vi "Send serial command.vi"(7 "Read?":bool, 8 "error IO":errorcluster, 10 "Send string":string=" 2 np", 11 "VISA resource name out":refnum<visa-resource-name>) -> (0 "error out":errorcluster={"status"=FALSE, "code"=1073676294, "source"="VISA Read in SMAC Parameters.vi->SMAC LabVIEW Toolkit_v1.vi"}, 2 "read string":string, 3 "VISA Out":refnum<visa-resource-name>)   [LabVIEW 2016]
panel:
  out "actual bytes read":u32
  out "Format String":string=" 1 03"
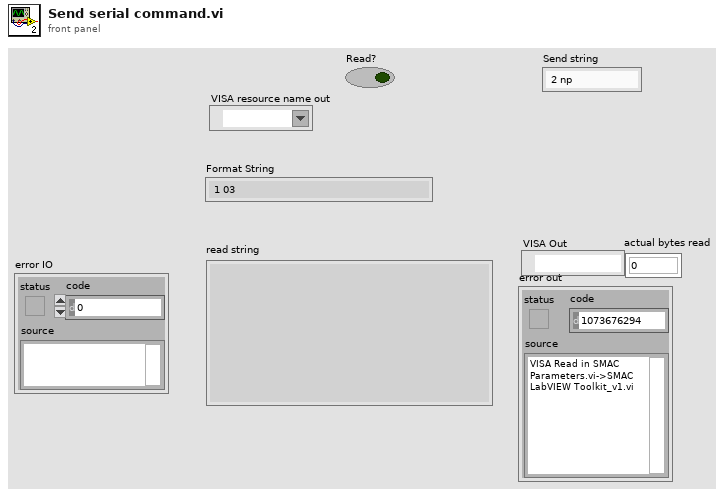
[diagram p1: front panel]
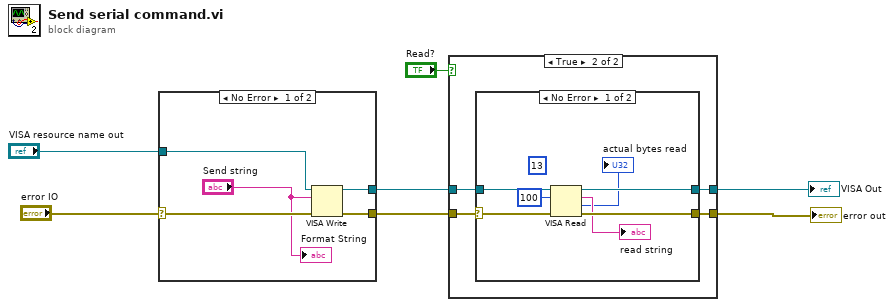
[diagram p0: block diagram]
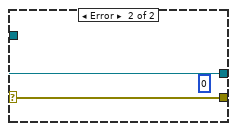
[diagram p4: hidden frame]
diagram:
  n1 = case shown="No Error" "error IO" {
    selector: "error IO" -> [w10 w14]
    tunnel: [w12 w13] -> w4
    tunnel: [w11 w14] -> w5
    tunnel: "VISA resource name out" -> [w8 w13]
    frame No Error {
      n2 = VISA Write(VISA resource name=w8, write buffer="Send string", error in (no error)=w10) -> (VISA resource name out=w12:refnum<visa-resource-name>, error out=w11:errorcluster)  [unwired: 1 out]
      "Format String" <- "Send string"
    }
    frame Error {
      (unwired) u32 0 ("return count")
    }
  }
  n3 = case shown="True" "Read?" {
    tunnel: w5 -> [w16 w20]
    tunnel: w4 -> [w15 w19]
    tunnel: [w15 w18] -> w3
    tunnel: [w16 w17] -> w2
    frame False {
    }
    frame True {
      n4 = case "Read bytes from port." shown="No Error" w20 {
        selector: w20 -> [w23 w28]
        tunnel: [w26 w28] -> w17
        tunnel: [w27 w29] -> w18
        tunnel: w19 -> [w24 w29]
        frame No Error {
          (unwired) u32 13 ("bytes to read")
          n5 = VISA Read(VISA resource name=w24, byte count=u32 100, error in (no error)=w23) -> (VISA resource name out=w27:refnum<visa-resource-name>, read buffer=→"read string":string, return count=→"actual bytes read":u32, error out=w26:errorcluster)
        }
        frame Error {
          # "Error occurred \nreading Bytes at \nSerial Port"
        }
      }
    }
  }
  "error out" <- w2
  "VISA Out" <- w3
